vi "error_cluster_from_error_code.vi"(4 "Cut first x elements\nfrom Error Chain (0)":i32, 5 "Is Warning (False)":bool, 6 "Error Creation Enabled (True)":bool=TRUE, 7 "Show Call Chain (True)":bool=TRUE, 8 "error in":errorcluster caption="error in (no error)", 9 "Error Message (\"\")":string, 10 "Error Enum in":T1=enum."VISA_err_Timeout", 11 "VISA resource name":refnum<visa-resource-name>) -> (0 "error out":errorcluster, 3 "VISA resource name out":refnum<visa-resource-name>)   [LabVIEW 2020, in "Rohde&Schwarz RTx Oscilloscopes.lvlib" / "rsidr_core.lvlib"]
uses:
  rsidr_core.lvlib
  type_Error_Codes.ctl
  _type_Operation_Fgv_Session.ctl
  Match Regular Expression.xnode
panel:
  out "Composed Error Source String":string
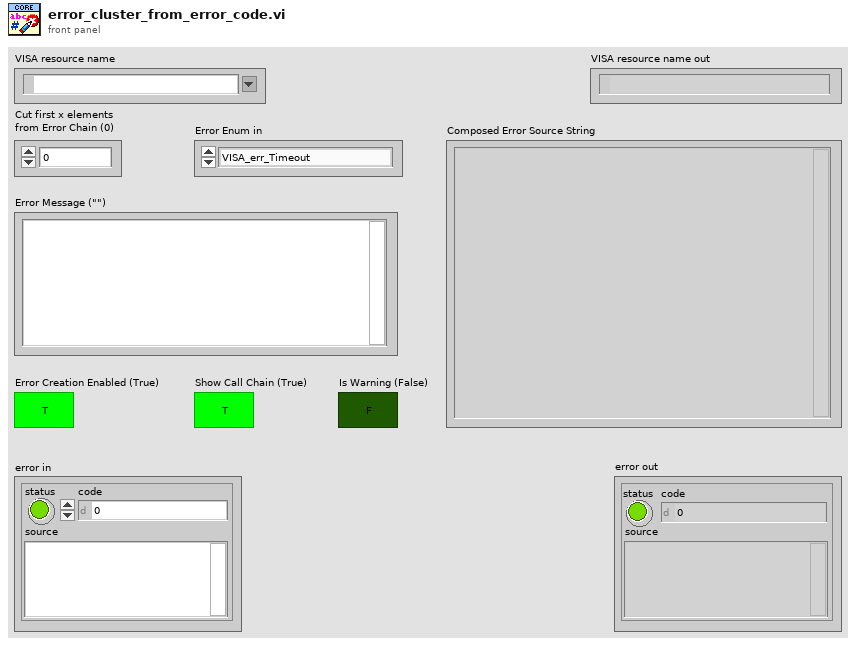
[diagram p1: front panel]
types:
  T1 = typedef "Rohde&Schwarz RTx Oscilloscopes.lvlib/rsidr_core.lvlib/type_Error_Codes.ctl" = enum16{"No_error", "VISA_err_ResourceNotFound", "VISA_err_Timeout", "VISA_warn_MoreDataAvailable", "RS_err_MissingCallback", "RS_err_InvalidAttribute", "RS_err_InvalidValue", "RS_err_UnknownResource", "RS_err_AlreadyInitialized", "RS_err_InstrumentStatus", "RS_err_BadRepCapName", "RS_err_TypesMismatch", "RS_err_ValueNotSupported", "RS_err_InvalidRngTable", "RS_err_IDqueryFail", "RS_err_UnexpResponse", "VISA_warn_ConfigNotLoaded", "RS_err_AttributeNotReadable", "RS_err_AttributeNotWritable", "RS_err_InstrumentType", "RS_err_InstrumentOption", "VISA_err_InvalidSize", "RS_err_ReliabilityIndicator", "VISA_warn_UnknownStatus", "VISA_warn_TermCharRead", "VISA_err_IO_error", "RS_err_FunctionNotSupported", "VISA_warn_QueueEmpty"}
  T2 = typedef "Rohde&Schwarz RTx Oscilloscopes.lvlib/rsidr_core.lvlib/_type_Operation_Fgv_Session.ctl" = enum16{"Initialize", "GetData", "SetData", "Clear", "GetSessionIx"}
  T3 = enum32{"invalid app kind", "Development System", "Run Time System", "Student Edition", "Embedded LabVIEW", "Evaluation", "Custom"}
  T4 = enum32{"invalid CPU target", "Motorola 68K", "PowerPC", "Intel x86", "SPARC", "PA-RISC", "MIPS", "Alpha", "ARM", "AMD/Intel x64"}
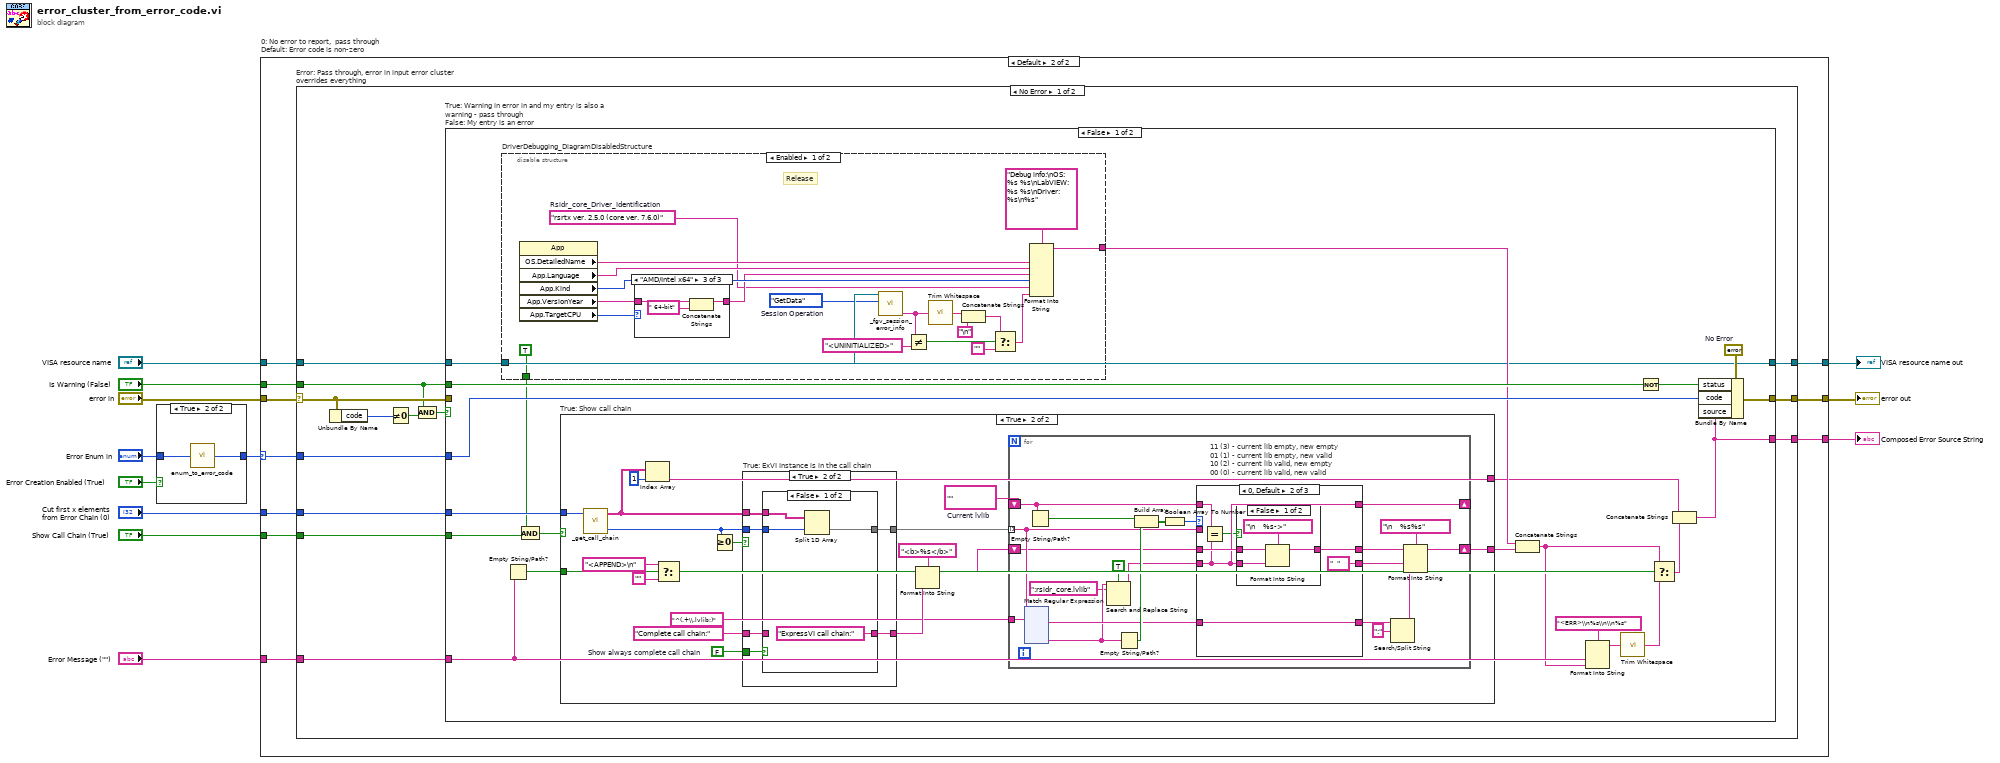
[diagram p0: block diagram]
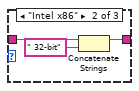
[diagram p5: hidden frame]
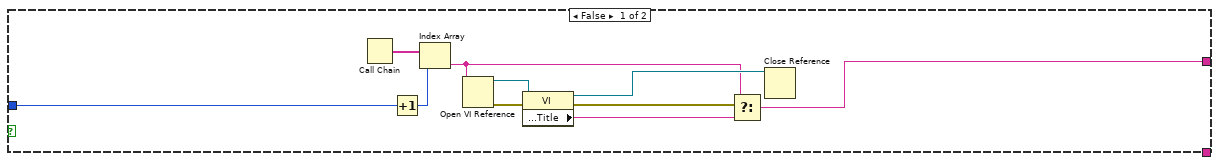
[diagram p7: hidden frame]
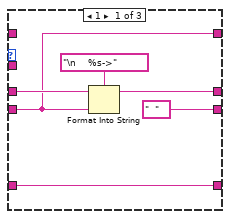
[diagram p8: hidden frame]
diagram:
  n1 = case shown="True" "Error Creation Enabled (True)" {
    tunnel: [_ w13] -> w10
    tunnel: "Error Enum in" -> [_ w14]
    frame False {
    }
    frame True {
      n2 = call "enum_to_error_code.vi"("Error Enum in"=w14) -> ("error code out"=w13:i32)  [unwired: 4 in]
    }
  }
  n3 = case "0: No error to report,  pass through\nDefault: Error code is non-zero" shown="Default" w10 {
    selector: w10 -> [_ w24]
    tunnel: [w16 w26] -> w12
    tunnel: "error in" -> [w16 w25]
    tunnel: [_ w23] -> w9
    tunnel: "VISA resource name" -> [w15 w22]
    tunnel: [w15 w21] -> w5
    tunnel: "Is Warning (False)" -> [_ w20]
    tunnel: "Cut first x elements\nfrom Error Chain (0)" -> [_ w19]
    tunnel: "Show Call Chain (True)" -> [_ w18]
    tunnel: "Error Message (\"\")" -> [_ w17]
    frame 0 {
    }
    frame Default {
      n4 = case "Error: Pass through, error in input error cluster overrides everything" shown="No Error" w25 {
        selector: w25 -> [w34 w288]
        tunnel: [w39 w288] -> w26
        tunnel: w24 -> [w38 _]
        tunnel: [w33 _] -> w23
        tunnel: w22 -> [w32 w287]
        tunnel: [w31 w287] -> w21
        tunnel: w20 -> [w30 _]
        tunnel: w19 -> [w29 _]
        tunnel: w18 -> [w28 _]
        tunnel: w17 -> [w27 _]
        frame No Error {
          n5 = Unbundle By Name(w34) -> ("code"=w37:i32)
          n6 = Not Equal To 0?(x=w37) -> (x != 0?=w35:bool)
          n7 = And(x=w30, y=w35) -> (x .and. y?=w36:bool)
          n8 = case "True: Warning in error in and my entry is also a warning - pass through\nFalse: My entry is an error" shown="False" w36 {
            tunnel: [w60 w286] -> w39
            tunnel: w38 -> [w58 _]
            tunnel: w34 -> [_ w286]
            tunnel: w30 -> [w57 _]
            tunnel: w27 -> [w55 _]
            tunnel: w28 -> [w47 _]
            tunnel: w29 -> [w51 _]
            tunnel: [w42 _] -> w33
            tunnel: w32 -> [w40 w285]
            tunnel: [w40 w285] -> w31
            frame False {
              w59 = errorcluster {"status"=FALSE, "code"=0, "source"=""}  # No Error
              n9 = disable-structure "DriverDebugging_DiagramDisabledStructure" shown="Enabled" {
                disable-tunnel: [w73 _] -> w44
                disable-tunnel: [TRUE _] -> w45
                disable-tunnel: w40 -> [w71 _]
                frame Enabled {
                  w61 = _type_Operation_Fgv_Session."GetData"  # Session Operation
                  w72 = "rsrtx ver. 2.5.0 (core ver. 7.6.0)"  # Rsidr_core_Driver_Identification
                  # "Release"
                  n10 = property on="Property Node" class="App"() -> ("OS.DetailedName"=w78:string, "App.Language"=w79:string, "App.Kind"=w80:T3, "App.VersionYear"=w77:string, "App.TargetCPU"=w76:T4)  [unwired: 2 in, 2 out]
                  n11 = case shown="\"AMD/Intel x64\"" w76 {
                    tunnel: w77 -> [w81 w84 w87]
                    tunnel: [w81 w82 w85] -> w75
                    frame Default {
                    }
                    frame "Intel x86" {
                      n12 = Concatenate Strings(w84, " 32-bit") -> (w82:string)
                    }
                    frame "AMD/Intel x64" {
                      n13 = Concatenate Strings(w87, " 64-bit") -> (w85:string)
                    }
                  }
                  n14 = call "_fgv_session_error_info.vi"("Operation"=w61, "Session in"=w71) -> ("Session Error Info out"=w67:string)  [unwired: 4 in, 1 out]
                  n15 = Not Equal?(x=w67, y="<UNINITIALIZED>" ("Session Error Info in (\"\")")) -> (x != y?=w69:bool)
                  n16 = call "Trim Whitespace.vi"("string"=w67) -> ("trimmed string"=w65:string)  [unwired: 1 in]
                  n17 = Concatenate Strings(w65, "\n") -> (w64:string)
                  n18 = Select(t=w64, s=w69, f="") -> (s? t:f=w66:string)
                  n19 = Format Into String(format string="Debug info:\nOS: %s %s\nLabVIEW: %s %s\nDriver: %s\n%s", w78, w79, w75, w80, w72, w66) -> (resulting string=w73:string)  [unwired: 2 in, 1 out]
                }
                frame Disabled {
                  # "Debug"
                }
              }
              n20 = Empty String/Path?(string/path=w55) -> (empty?=w50:bool)
              n21 = Compound Arithmetic op=AND(w45, w47) -> (w46:bool)
              n22 = case "True: Show call chain" shown="True" w46 {
                tunnel: [_ w105] -> w49
                tunnel: w50 -> [_ w116]
                tunnel: w51 -> [w96 w104]
                tunnel: [w88 w99] -> w43
                frame False {
                  n23 = Call Chain() -> (call chain=w97:string[])
                  n24 = Increment(x=w96) -> (x+1=w95:i32)
                  n25 = Index Array(array=w97, index=w95) -> (element=w89:string)
                  n26 = Open VI Reference(vi path=w89) -> (vi reference=w94:refnum<vi>, error out=w90:errorcluster)  [unwired: 5 in]
                  n27 = property on="Property Node" class="VI"(reference=w94, error in=w90) -> (reference out=w93:refnum<vi>, error out=w91:errorcluster, "Front Panel Window:Title"=w92:string)
                  n28 = Select(t=w89, s=w91, f=w92) -> (s? t:f=w88:string)
                  n29 = Close Reference(reference=w93) -> ()  [unwired: 1 in, 1 out]
                }
                frame True {
                  w109 = ""  # Current lvlib
                  w113 = FALSE  # Show always complete call chain
                  n30 = call "_get_call_chain.vi"("Cut first x elements\nfrom Error Chain (0)"=w104) -> ("ExVI index out"=w101:i32, "Call chain out"=w102:string[])  [unwired: 2 in, 1 out]
                  n31 = Index Array(array=w102, index=1) -> (element=w99:string)
                  n32 = Select(t="<APPEND>\n", s=w116, f="" ("Empty String Constant")) -> (s? t:f=w98:string)
                  n33 = Greater Or Equal To 0?(x=w101) -> (x >= 0?=w100:bool)
                  n34 = case "True: ExVI Instance is in the call chain" shown="True" w100 {
                    tunnel: [w271 w278] -> w108
                    tunnel: w113 -> [_ w277]
                    tunnel: "Complete call chain:" ("call chain header") -> [w272 w276]
                    tunnel: [w272 w275] -> w107
                    tunnel: w102 -> [w271 w274]
                    tunnel: w101 -> [_ w273]
                    frame False {
                    }
                    frame True {
                      n35 = case shown="False" w277 {
                        tunnel: w274 -> [w279 w283]
                        tunnel: w273 -> [w280 _]
                        tunnel: [w281 w283] -> w278
                        tunnel: ["ExpressVI call chain:" ("call chain header") w284] -> w275
                        tunnel: w276 -> [_ w284]
                        frame False {
                          n36 = Split 1D Array(array=w279, index=w280) -> (second subarray=w281:string[])  [unwired: 1 out]
                        }
                        frame True {
                        }
                      }
                    }
                  }
                  n37 = Format Into String(format string="<b>%s</b>", initial string=w98, w107) -> (resulting string=w111:string)  [unwired: 1 in, 1 out]
                  n38 = for {
                    tunnel: w108 -> [w131] mode=indexing
                    shift-right: [w127] -> w105
                    shift-left: w111 -> [w126]
                    tunnel: "^(.+\\.lvlib:)" ("search string/char (-)") -> [w137]
                    shift-right: [w130] -> _
                    shift-left: w109 -> [w136]
                    n39 = xnode ("Match Regular Expression")("input string"=w131, "regular expression"=w137) -> ("after match"=w132:string, "submatch 1"=w120:string)  [unwired: 4 in, 4 out]
                    n40 = Empty String/Path?(string/path=w136) -> (empty?=w135:bool)
                    n41 = Search and Replace String(case sensitive?=TRUE ("ignore case? (F)"), input string=w120, search string=":rsidr_core.lvlib") -> (result string=w117:string)  [unwired: 5 in, 3 out]
                    n42 = Empty String/Path?(string/path=w120) -> (empty?=w134:bool)
                    n43 = Build Array(w135, w134) -> (w133:bool[])
                    n44 = Boolean Array To Number(Boolean array=w133) -> (number=w123:u32)
                    n45 = case "11 (3) - current lib empty, new empty\n01 (1) - current lib empty, new valid\n10 (2) - current lib valid, new empty\n00 (0) - current lib valid, new valid" shown="0, Default" w123 {
                      tunnel: w136 -> [_ w146 _]
                      tunnel: w132 -> [w139 w148 _]
                      tunnel: w131 -> [_ _ w156]
                      tunnel: [w138 w147 _] -> w130
                      tunnel: ["  " "  " _] -> w122
                      tunnel: [w139 w148 w156] -> w128
                      tunnel: w126 -> [w142 w150 w157]
                      tunnel: [w141 w149 w157] -> w125
                      tunnel: w117 -> [w138 w147 _]
                      frame 1 {
                        n46 = Format Into String(format string="\n    %s->", initial string=w142, w138) -> (resulting string=w141:string)  [unwired: 1 in, 1 out]
                      }
                      frame 0, Default {
                        n47 = Equal?(x=w146, y=w147) -> (x = y?=w145:bool)
                        n48 = case shown="False" w145 {
                          tunnel: w150 -> [w154 w155]
                          tunnel: [w153 w155] -> w149
                          tunnel: w147 -> [w151 _]
                          frame False {
                            n49 = Format Into String(format string="\n    %s->", initial string=w154, w151) -> (resulting string=w153:string)  [unwired: 1 in, 1 out]
                          }
                          frame True {
                          }
                        }
                      }
                      frame 2, 3 {
                      }
                    }
                    n50 = Search/Split String(string=w128, search string/char (-)=":") -> (substring before match=w121:string)  [unwired: 1 in, 2 out]
                    n51 = Format Into String(format string="\n    %s%s", initial string=w125, w122, w121) -> (resulting string=w127:string)  [unwired: 1 in, 1 out]
                  }
                }
              }
              n52 = Concatenate Strings(w44, w49) -> (w48:string)
              n53 = Format Into String(format string="<ERR>\\n%s\\n\\n%s", w55, w48) -> (resulting string=w54:string)  [unwired: 2 in, 1 out]
              n54 = call "Trim Whitespace.vi"("string"=w54) -> ("trimmed string"=w41:string)  [unwired: 1 in]
              n55 = Not(x=w57) -> (.not. x?=w52:bool)
              n56 = Select(t=w48, s=w50, f=w41) -> (s? t:f=w53:string)
              n57 = Concatenate Strings(w43, w53) -> (w42:string)
              n58 = Bundle By Name(cluster=w59, "status"=w52, "code"=w58, "source"=w42) -> (w60:errorcluster)
            }
            frame True {
            }
          }
        }
        frame Error {
        }
      }
    }
  }
  "error out" <- w12
  "Composed Error Source String" <- w9
  "VISA resource name out" <- w5
